vi "Identify.vi"(0 "VISA resource name":refnum<visa-resource-name>, 11 "error in (no error)":errorcluster) -> (4 "VISA resource name out":refnum<visa-resource-name>, 8 "Identity":string, 15 "error out":errorcluster)   [LabVIEW 2023, in "ACM Visa Driver.lvlib"]
uses:
  ACM Visa Driver.lvlib
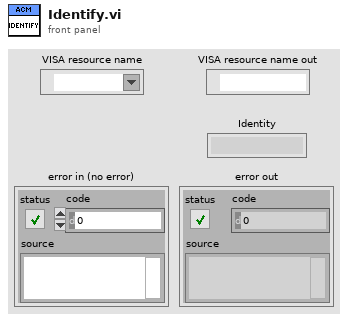
[diagram p1: front panel]
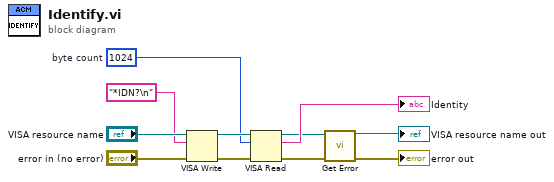
[diagram p0: block diagram]
diagram:
  w4 = u32 1024  # byte count
  n1 = VISA Write(VISA resource name="VISA resource name", write buffer="*IDN?\n", error in (no error)="error in (no error)") -> (VISA resource name out=w8:refnum<visa-resource-name>, error out=w7:errorcluster)  [unwired: 1 out]
  n2 = VISA Read(VISA resource name=w8, byte count=w4, error in (no error)=w7) -> (VISA resource name out=w2:refnum<visa-resource-name>, read buffer=→"Identity":string, error out=w6:errorcluster)  [unwired: 1 out]
  n3 = call "Get Error.vi"("VISA resource name"=w2, "error in (no error)"=w6) -> ("VISA resource name out"=→"VISA resource name out":refnum<visa-resource-name>, "error out"=→"error out":errorcluster)  [unwired: 12 in]
